vi "USRP Send Software Start Trigger.vi"(0 "niUsrpRio Session":T1={"FPGA Interface"=refnum, "RIO Interface Number"=0, "Data Clock Rate"=0, "FPGA Data Clock Rate"=0, "Global Settings Register Bus"=refnum, "Radio 0 Settings Register Bus"=refnum, "Radio 1 Settings Register Bus"=refnum, "Radio Settings Bus Semaphore"=refnum, "DB Queues"=[], "Characterization Data Valid?"=FALSE, "EEPROM Header"={"Checksum"=0, "Product Code"=0, "Hardware Current Version"=0, "Hardware Oldest Compatible Version"=0, "EEPROM Map Current Version"=0, "EEPROM Map Oldest Compatible Version"=0, "User Password"="", "Pointer to Factory Header"=0, "Pointer to User Header"=0, "Recommended Interval"=0, "Number of Reserved Bytes"=9, "Number of Daughterboards"=0, "Daughterboard IDs"=[], "Daughterboard Serial Numbers"=[]}, "Device Data Header"={"Checksum"=0, "Number of Channels"=0, "Number of Gain Settings"=[], "Pointer to Characterization Data"=[], "Number of Reserved Bytes"=27, "Number of Frequencies"=[]}, "EEPROM Characterization Header"={"Checksum"=0, "Date"=timestamp(0 s since 1904-01-01), "Temperature"=0.0, "Misc. Info"="", "Pointer to Device Data Header"=0, "Number of Reserved Bytes"=28}, "Characterization Data"=[], "FPGA Current Version"=0, "FPGA Oldest Compatible Version"=0, "Fixed Logic Current Version"=0, "Fixed Logic Oldest Compatible Version"=0, "FPGA Radio Settings Bus Current Version"=0, "FPGA Radio Settings Bus Oldest Compatible Version"=0, "FPGA Board Config Current Version"=0, "FPGA Board Config Oldest Compatible Version"=0, "Daughterboard Clock Rate"=0, "daughterboard configuration session handles"=[]} {"Daughterboard Clock Rate" format="%#.3pHz"; "FPGA Data Clock Rate" format="%#.3pHz"; "Data Clock Rate" format="%#.3pHz"; "Characterization Data"."Frequencies [Hz]" format="%#_6p"; "EEPROM Characterization Header"."Pointer to Device Data Header" format="%x"; "EEPROM Characterization Header"."Checksum" format="%x"; "Device Data Header"."Pointer to Characterization Data" format="%x"; "Device Data Header"."Checksum" format="%x"; "EEPROM Header"."Pointer to User Header" format="%x"; "EEPROM Header"."Pointer to Factory Header" format="%x"; "EEPROM Header"."Product Code" format="%x"; "EEPROM Header"."Checksum" format="%x"}, 1 "scope":string(combo)="rx", 11 "error in":errorcluster) -> (4 "niUsrpRio Session (out)":T1={"FPGA Interface"=refnum, "RIO Interface Number"=0, "Data Clock Rate"=0, "FPGA Data Clock Rate"=0, "Global Settings Register Bus"=refnum, "Radio 0 Settings Register Bus"=refnum, "Radio 1 Settings Register Bus"=refnum, "Radio Settings Bus Semaphore"=refnum, "DB Queues"=[], "Characterization Data Valid?"=FALSE, "EEPROM Header"={"Checksum"=0, "Product Code"=0, "Hardware Current Version"=0, "Hardware Oldest Compatible Version"=0, "EEPROM Map Current Version"=0, "EEPROM Map Oldest Compatible Version"=0, "User Password"="", "Pointer to Factory Header"=0, "Pointer to User Header"=0, "Recommended Interval"=0, "Number of Reserved Bytes"=9, "Number of Daughterboards"=0, "Daughterboard IDs"=[], "Daughterboard Serial Numbers"=[]}, "Device Data Header"={"Checksum"=0, "Number of Channels"=0, "Number of Gain Settings"=[], "Pointer to Characterization Data"=[], "Number of Reserved Bytes"=27, "Number of Frequencies"=[]}, "EEPROM Characterization Header"={"Checksum"=0, "Date"=timestamp(0 s since 1904-01-01), "Temperature"=0.0, "Misc. Info"="", "Pointer to Device Data Header"=0, "Number of Reserved Bytes"=28}, "Characterization Data"=[], "FPGA Current Version"=0, "FPGA Oldest Compatible Version"=0, "Fixed Logic Current Version"=0, "Fixed Logic Oldest Compatible Version"=0, "FPGA Radio Settings Bus Current Version"=0, "FPGA Radio Settings Bus Oldest Compatible Version"=0, "FPGA Board Config Current Version"=0, "FPGA Board Config Oldest Compatible Version"=0, "Daughterboard Clock Rate"=0, "daughterboard configuration session handles"=[]} {"Daughterboard Clock Rate" format="%#.3pHz"; "FPGA Data Clock Rate" format="%#.3pHz"; "Data Clock Rate" format="%#.3pHz"; "Characterization Data"."Frequencies [Hz]" format="%#_6p"; "EEPROM Characterization Header"."Pointer to Device Data Header" format="%x"; "EEPROM Characterization Header"."Checksum" format="%x"; "Device Data Header"."Pointer to Characterization Data" format="%x"; "Device Data Header"."Checksum" format="%x"; "EEPROM Header"."Pointer to User Header" format="%x"; "EEPROM Header"."Pointer to Factory Header" format="%x"; "EEPROM Header"."Product Code" format="%x"; "EEPROM Header"."Checksum" format="%x"}, 15 "error out":errorcluster)   [LabVIEW 2016]
doc: "Sends a software Start Trigger to the device.\n\n<B>Input Parameters</B>\n\n<B>niUsrpRio Session</B> is the object created by the Open VI and used as the session handle for the USRP RIO design library.\n\n<B>scope</B> is the channel on which software trigger is to be sent. The options are \"rx/RF 0\", \"rx/RF 1\", \"tx/RF 0\", and \"tx/RF 1\".\n\n<B>error in</B> describes error conditions that occur before this node runs. This input provides standard 'error in' functionality.\n\n<B>Output Parameters</B>\n\n<B>niUsrpRio Session (out)</B> is the niUsrpRio session used in all subsequent USRP RIO design library host VIs.\n\n<B>error out</B> contains error information. This output provides standard 'error out' functionality."
uses:
  <instrlib>/niUsrpRio/Config/v1/Host/Public/niUsrpRio Session.ctl
  <instrlib>/_niInstr/Register Bus/v0/Host/Public/Register Bus Session.ctl
  <instrlib>/_niInstr/Register Bus/v0/Host/Private/Session Data.ctl
  <instrlib>/niUsrpRio/Config/v1/Host/Private/DB Queue Reference.ctl
  <instrlib>/niUsrpRio/Config/v1/Host/Private/Daughterboard Data.ctl
  <instrlib>/niUsrpRio/Config/v1/Host/Private/ATR state data.ctl
  <instrlib>/niUsrpRio/Config/v1/Host/Private/Antenna Configuration.ctl
  <instrlib>/niUsrpRio/Config/v1/Host/Private/CPLD Power Mode.ctl
  <instrlib>/niUsrpRio/Config/v1/Host/Public/EEPROM Header.ctl
  <instrlib>/niUsrpRio/Config/v1/Host/Public/EEPROM Device Data Header.ctl
  <instrlib>/niUsrpRio/Config/v1/Host/Public/EEPROM Characterization Header.ctl
  <instrlib>/niUsrpRio/Config/v1/Host/Public/Characterization Data.ctl
  <instrlib>/niUsrpRio/Config/v1/Host/Public/IQ Imbalance.ctl
  USRP Streaming Xvcr FPGA Ref.ctl
  <vilib>/rvi/errors/niLvFpgaAdjustHostInterfaceError.vi
  <vilib>/Utility/error.llb/Error Cluster From Error Code.vi
  <vilib>/rvi/interface/nirviReadWriteControl/nirviReadWriteControl.xnode
  <vilib>/rvi/interface/Simulation/niFpgaSimulationCallBeginRW.vi
  NiFpgaLv.dll
  <instrlib>/niUsrpRio/Config/v1/Host/niUsrpRio Config v1 Host.lvlib
  <instrlib>/_niInstr/Register Bus/v0/Host/niInstr Register Bus v0 Host.lvlib
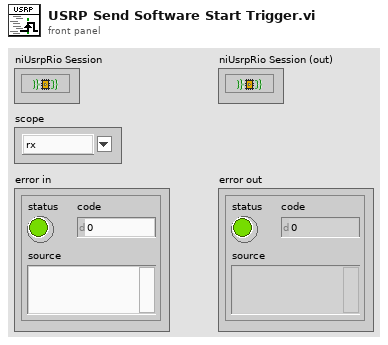
[diagram p1: front panel]
types:
  T1 = typedef "niUsrpRio Config v1 Host.lvlib/niUsrpRio Session.ctl" = cluster{"FPGA Interface":refnum<k20>, "RIO Interface Number":u32, "Data Clock Rate":u32, "FPGA Data Clock Rate":u32, "Global Settings Register Bus":T2, "Radio 0 Settings Register Bus":T2, "Radio 1 Settings Register Bus":T2, "Radio Settings Bus Semaphore":T3, "DB Queues":T4[], "Characterization Data Valid?":bool, "EEPROM Header":T5, "Device Data Header":T6, "EEPROM Characterization Header":T7, "Characterization Data":T8[], "FPGA Current Version":u32, "FPGA Oldest Compatible Version":u32, "Fixed Logic Current Version":u32, "Fixed Logic Oldest Compatible Version":u32, "FPGA Radio Settings Bus Current Version":u32, "FPGA Radio Settings Bus Oldest Compatible Version":u32, "FPGA Board Config Current Version":u32, "FPGA Board Config Oldest Compatible Version":u32, "Daughterboard Clock Rate":u32, "daughterboard configuration session handles":u64[]}
  T2 = typedef "niInstr Register Bus v0 Host.lvlib/Register Bus Session.ctl" = refnum<queue>
  T3 = typedef "Semaphore RefNum" = refnum<k1>
  T4 = typedef "niUsrpRio Config v1 Host.lvlib/DB Queue Reference.ctl" = refnum<queue>
  T5 = typedef "niUsrpRio Config v1 Host.lvlib/EEPROM Header.ctl" = cluster{"Checksum":u32, "Product Code":u16, "Hardware Current Version":u16, "Hardware Oldest Compatible Version":u16, "EEPROM Map Current Version":u16, "EEPROM Map Oldest Compatible Version":u16, "User Password":string, "Pointer to Factory Header":u32, "Pointer to User Header":u32, "Recommended Interval":u16, "Number of Reserved Bytes":i32, "Number of Daughterboards":u8, "Daughterboard IDs":u16[], "Daughterboard Serial Numbers":string[]}
  T6 = typedef "niUsrpRio Config v1 Host.lvlib/EEPROM Device Data Header.ctl" = cluster{"Checksum":u32, "Number of Channels":u8, "Number of Gain Settings":u16[], "Pointer to Characterization Data":u32[], "Number of Reserved Bytes":i32, "Number of Frequencies":u16[]}
  T7 = typedef "niUsrpRio Config v1 Host.lvlib/EEPROM Characterization Header.ctl" = cluster{"Checksum":u32, "Date":timestamp, "Temperature":sgl, "Misc. Info":string, "Pointer to Device Data Header":u32, "Number of Reserved Bytes":i32}
  T8 = typedef "niUsrpRio Config v1 Host.lvlib/Characterization Data.ctl" = cluster{"Gains[dB]":dbl[], "Frequencies [Hz]":dbl[], "IQ Imbalance Table":T9[], "Measured Gains[dB]":dbl[][]}
  T9 = typedef "niUsrpRio Config v1 Host.lvlib/IQ Imbalance.ctl" = cluster{"Gain Imbalance [linear]":dbl, "Phase Imbalance [radians]":dbl, "Offset":cdb}
  T10 = typedef "USRP Streaming Xvcr FPGA Ref.ctl" = refnum<k20>
  T11 = typedef "niUsrpRio Config v1 Host.lvlib/Device Subfunction.ctl" = enum16{"rx", "tx", "all"}
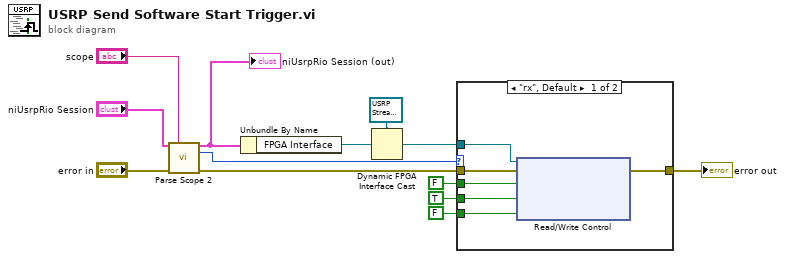
[diagram p0: block diagram]
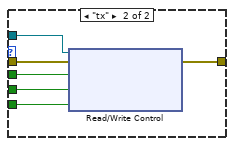
[diagram p2: hidden frame]
diagram:
  n1 = call <instrlib>:"Parse Scope 2.vi"("niUsrpRio Session"="niUsrpRio Session", "scope"="scope", "error in"="error in") -> ("niUsrpRio Session (out)"=w4:T1, "Device Subfunction"=w5:T11, "error out"=w8:errorcluster)  [unwired: 4 in, 6 out]
  "niUsrpRio Session (out)" <- w4
  n2 = Unbundle By Name(w4) -> ("FPGA Interface"=w2:refnum<k20>)
  n3 = Dynamic FPGA Interface Cast(Session In=T10 refnum ("FPGA VI Reference Out"), Type=w2) -> (Session Out=w1:T10)
  n4 = case shown="\"rx\", Default" w5 {
    tunnel: [w19 w25] -> w13
    tunnel: w1 -> [w14 w20]
    tunnel: w8 -> [w18 w24]
    tunnel: FALSE ("rf in.sw start trigger") -> [w17 w23]
    tunnel: TRUE ("rf in.sw start trigger") -> [w16 w22]
    tunnel: FALSE ("rf in.sw start trigger") -> [w15 w21]
    frame "rx", Default {
      n5 = xnode "Read/Write Control"("FPGA VI Reference In"=w14, "error in"=w18, "rx.software trigger"=w17, "rx.software trigger"=w16, "rx.software trigger"=w15) -> ("error out"=w19:errorcluster)  [unwired: 1 out]
    }
    frame "tx" {
      n6 = xnode "Read/Write Control"("FPGA VI Reference In"=w20, "error in"=w24, "tx.software trigger"=w23, "tx.software trigger"=w22, "tx.software trigger"=w21) -> ("error out"=w25:errorcluster)  [unwired: 1 out]
    }
  }
  "error out" <- w13
